vi "Write DAQ Control.vi"(8 "error in (no error)":errorcluster, 10 "DAQ Control":T1, 11 "Monkey in":refnum<class "Monkey.lvclass">) -> (0 "error out":errorcluster, 3 "Monkey out":refnum<class "Monkey.lvclass">)   [LabVIEW 2020, in "Monkey.lvlib" / "Monkey.lvclass"]
uses:
  Monkey.lvclass
  Run Utilities/TypeDefs/DAQ Control.ctl
  Monkey.lvclass/Monkey.ctl
  Run Utilities/Run Utilities.lvlib
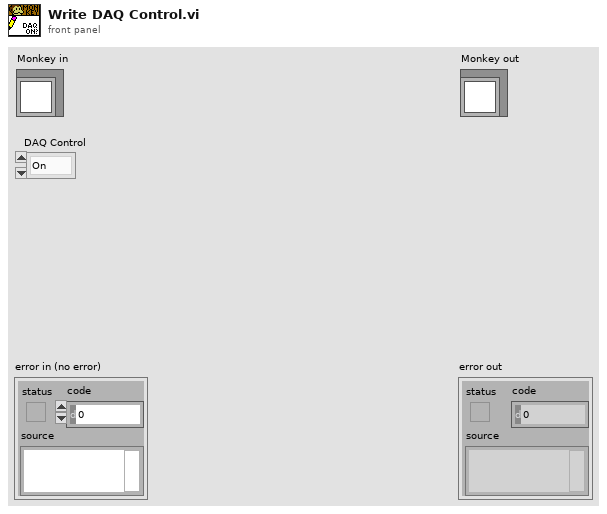
[diagram p1: front panel]
types:
  T1 = typedef "TALOS.lvlib/Run Utilities.lvlib/DAQ Control.ctl" = enum16{"On", "Off", "External"}
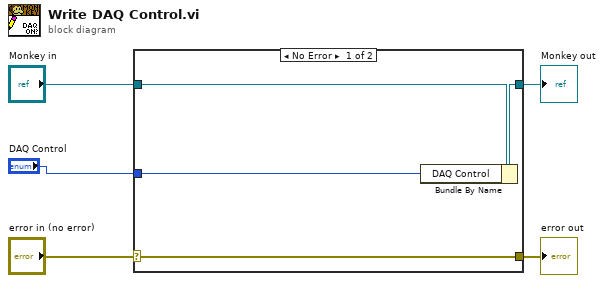
[diagram p0: block diagram]
diagram:
  n1 = case shown="No Error" "error in (no error)" {
    selector: "error in (no error)" -> [w9 w10]
    tunnel: [w9 w10] -> w4
    tunnel: [w7 w11] -> w2
    tunnel: "Monkey in" -> [w8 w11]
    tunnel: "DAQ Control" -> [w6 _]
    frame No Error {
      n2 = Bundle By Name(cluster=w8, "DAQ Control"=w6) -> (w7:refnum<class "Monkey.lvclass">)
    }
    frame Error {
    }
  }
  "error out" <- w4
  "Monkey out" <- w2
